vi "SwerveDrivePoseEst_VisionCorrect_Kalman_H_Callback.vi"(9 "U":T1, 10 "X":T1, 11 "ExtraPassedData":variant) -> (0 "Error":bool, 3 "Result":T1)   [LabVIEW 2019, in "Trajectory_Library.lvlib"]
doc: "Swerve Drive Pose Estimator, Kalman Filter H function for vision correction. This function passes the X matrix to the resulting matrix. No calculations are done.\n\nInput:\n - ExtraPassedData -- Variant contaiing extra data for the callback For this function the extra data should be empty..\n - X Matrix -- X matrix\n - U Matrix -- U matrix\n\nOutput:\n - Result -- Matrix resulting from calculation\n - Error -- If TRUE an error occured"
uses:
  Trajectory_Library.lvlib
  <vilib>/Analysis/Matrix/Datatypes/RealMatrix.ctl
  <vilib>/Analysis/Matrix/NI_Matrix.lvlib
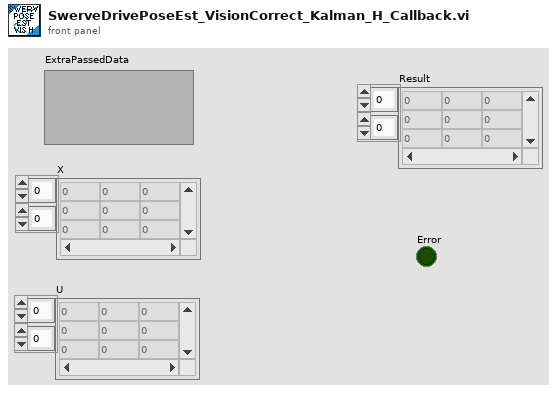
[diagram p1: front panel]
types:
  T1 = typedef "NI_Matrix.lvlib/RealMatrix.ctl" = dbl[][]
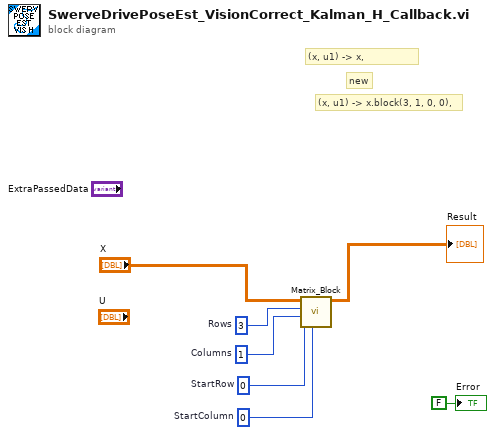
[diagram p0: block diagram]
diagram:
  w2 = 3  # Rows
  w3 = 1  # Columns
  w4 = 0  # StartRow
  w5 = 0  # StartColumn
  # "(x, u1) -> x.block(3, 1, 0, 0),"
  # "new"
  # "(x, u1) -> x,"
  n1 = call "Matrix_Block.vi"("StartColumn"=w5, "StartRow"=w4, "Columns"=w3, "Rows"=w2, "input matrix"="X") -> ("output matrix"=→"Result":T1)  [unwired: 6 in]
  "Error" <- FALSE ("Error")
